vi "RotateRight.vi"   [LabVIEW 2016, in "LineFollower2Sensor.lvrbt"]
uses:
  LineFollower2Sensor.lvrbt
  <vilib>/NXT/Hardware/Plugins/Tetrix DC Motor/TetrixDCMotorAddress.ctl
  <vilib>/NXT/NXTIO Xnodes/NXTIONodeSubVIs/TETRIX IO Move DC Motors.vi
  <vilib>/NXT/NXTIO Xnodes/NXTIONodeSubVIs/TETRIX IO Stop DC Motors.vi
  <vilib>/NXT/Subs/LVHSConnector.ctl
  <vilib>/NXT/NXTIO Xnodes/AddressXNode/NXTIOAddress.xnode
  <vilib>/NXT/NXTIO Xnodes/NXTIOXNode/NXTIO.xnode
  <vilib>/NXT/LegoClasses/BrickReference/BrickReference.lvclass
types:
  T1 = typedef "TetrixDCMotorAddress.ctl" = i32
  T2 = typedef "LVHSConnector.ctl" = refnum<class "BrickReference.lvclass">
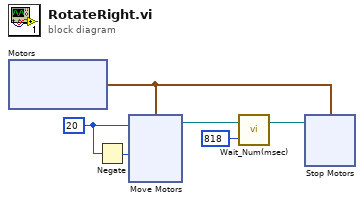
[diagram p0: block diagram]
diagram:
  w1 = i8 20 ("Power/Speed 1")
  n1 = xnode "Motors"() -> ("Motor"=w3:cluster{"TetrixDCMotor":T1, "TetrixDCMotor":T1})
  n2 = Negate(x=w1) -> (-x=w2:i8)
  n3 = xnode "Move Motors"("Power/Speed 2"=w2, "Power/Speed 1"=w1, "Motors"=w3) -> ("NXT/EV3"=w6:T2)  [unwired: 1 in]
  n4 = call <vilib>:"Wait_Num(msec).vi"("Time (100 msec)"=u32 818, "NXT/EV3"=w6) -> ("NXT/EV3"=w4:T2)  [unwired: 2 in]
  n5 = xnode "Stop Motors"("Motors"=w3, "NXT/EV3"=w4) -> ()  [unwired: 1 out]
